vi "String_Boolean to OnOff string.vi"(3 "Boolean value":bool) -> (1 "ON/OFF string":string)   [LabVIEW 2020]
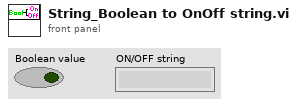
[diagram p1: front panel]
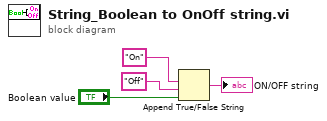
[diagram p0: block diagram]
diagram:
  n1 = Append True/False String(1:"Boolean value", 2:"Off" ("false string"), 3:"On" ("true string")) -> (0:→"ON/OFF string":string)  [unwired: 1 in]
